vi "align single wall angleV1.0.vi"(8 "error in (no error)":errorcluster, 9 "gyro degree":dbl, 10 "dir":bool, 11 "Target Voltage":dbl) -> (0 "Error Out":errorcluster)   [LabVIEW 2019]
uses:
  <vilib>/Platform/TimedLoop/XDataNode/timing_clust.ctl
  <vilib>/Platform/TimedLoop/XDataNode/nitl_modes.ctl
  <vilib>/Platform/TimedLoop/XDataNode/wakeup.ctl
  <vilib>/addons/control/pid/pid.llb/PID (DBL).vi
  <vilib>/platform/TimedLoop/XDataNode/XDataNode.xnode
  <vilib>/Platform/TimedLoop/XDataNode/XDNodeRunTimeDep.lvlib
  <vilib>/addons/control/pid/NI_PID_pid.lvlib
panel:
  out "Waveform Chart 2":dbl(graph)
  out "Waveform Chart":dbl(graph)
  in  "skip IR":bool
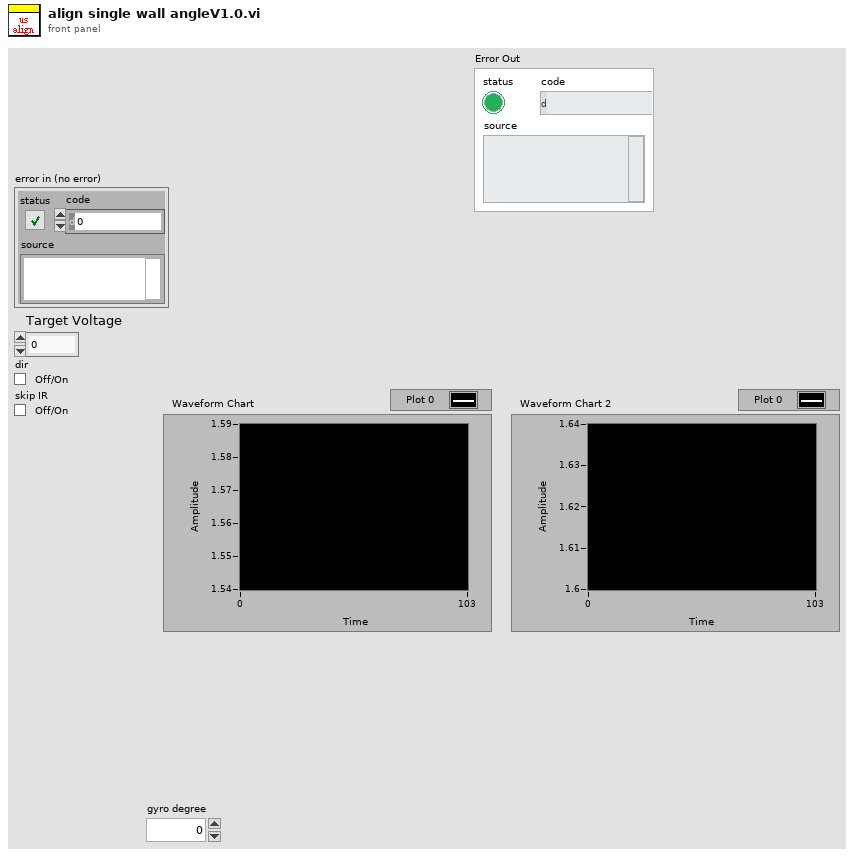
[diagram p1: front panel]
types:
  T1 = typedef "XDNodeRunTimeDep.lvlib/timing_clust.ctl" = cluster{"Expected End [f-1]":u64, "Actual End [f-1]":u64, "Finished Late? [f-1]":bool, "Expected End [i-1]":u64, "Actual End [i-1]":u64, "Finished Late? [i-1]":bool, "Expected Start [i]":u64, "Actual Start [i]":u64, "Expected Start [f]":u64, "Actual Start [f]":u64, "Source Name":string, "Structure Name":string, "Period":i64, "Deadline":i64, "Offset":i64, "Start":i64, "Priority":i32, "Timeout":i32, "Mode":T2, "Wakeup Reason":T3, "Error":errorcluster, "Source Type":string, "Secondary Source Type":string, "Global End Time":u64, "Global Start Time":u64, "Frame Duration":u64, "Iteration Duration":u64, "Assigned CPU":i32, "I/O Scan Engine Mode":u32}
  T2 = typedef "XDNodeRunTimeDep.lvlib/nitl_modes.ctl" = enum32{"No Change", "Process missed periods, maintain original phase", "Discard missed periods, maintain original phase", "Process missed periods, ignore original phase", "Discard missed periods, ignore original phase"}
  T3 = typedef "XDNodeRunTimeDep.lvlib/wakeup.ctl" = enum32{"Normal", "Aborted", "Asynchronous wakeup", "Timing source error", "Timed loop error", "Timeout"}
  T4 = typedef "IR out.ctl" = cluster{"DC estimate (V) 2":dbl, "DC estimate (V)":dbl, "AC estimate (Vrms)":dbl, "AC estimate (Vrms) 2":dbl}
  T5 = cluster{"dbl Scaled Value":dbl, "dbl Scaled Value":dbl}
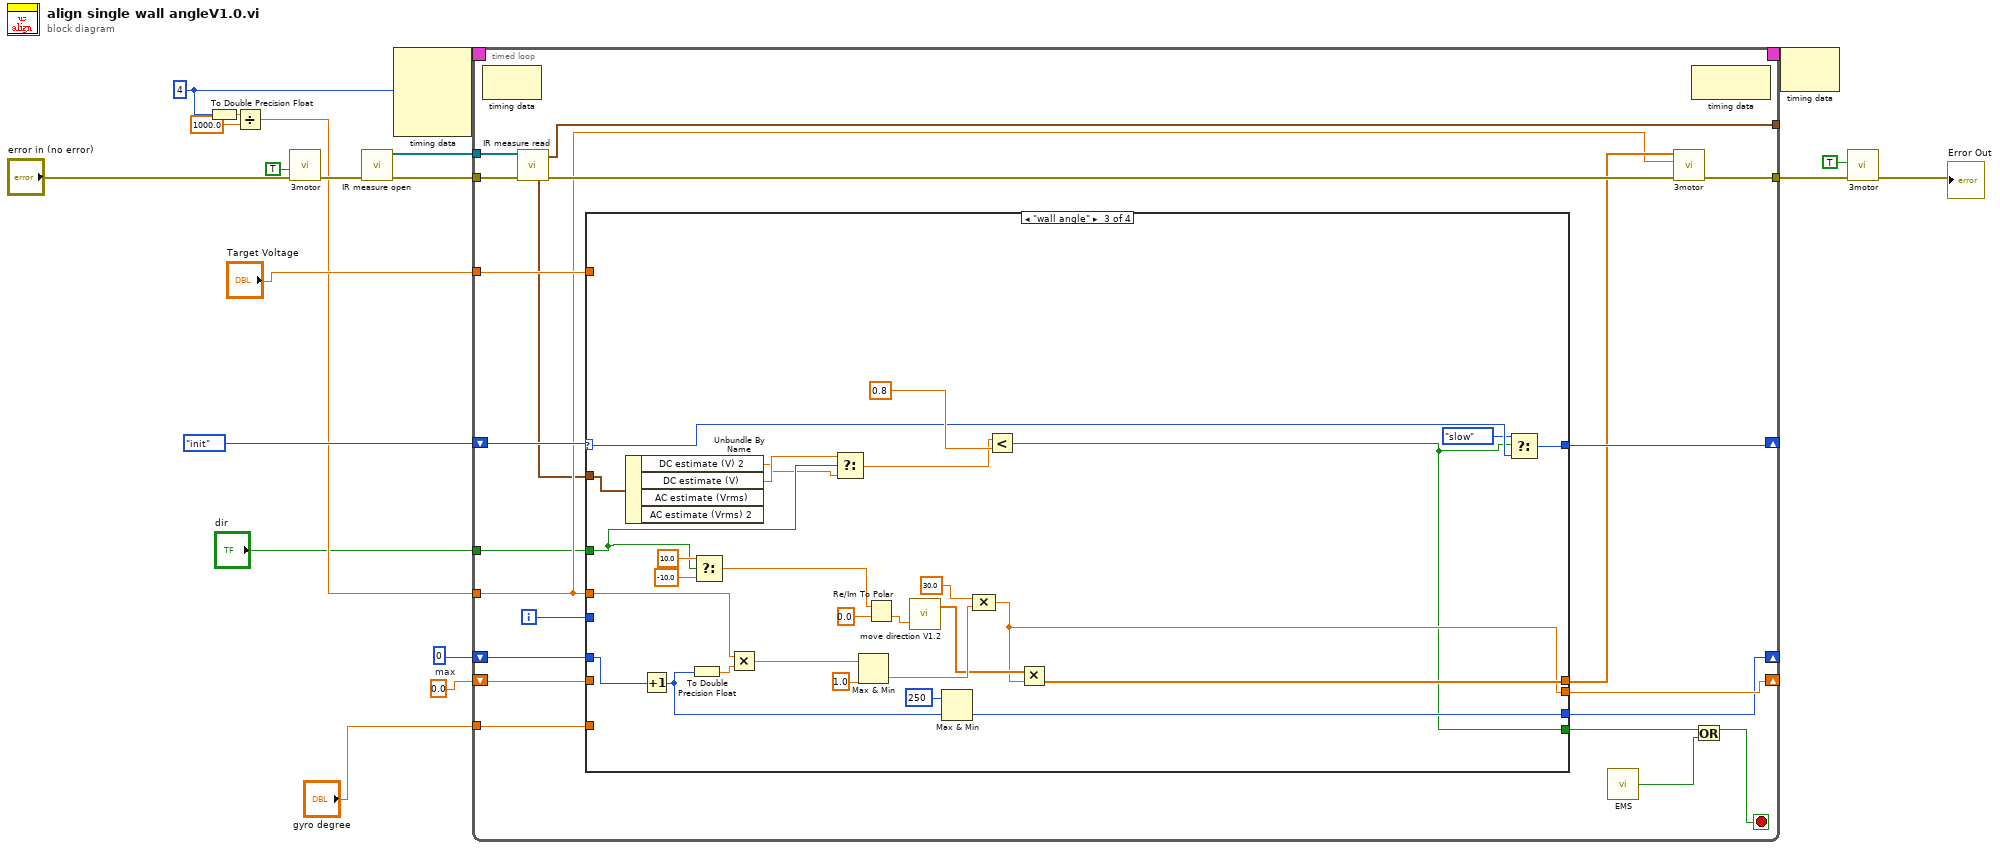
[diagram p0: block diagram]
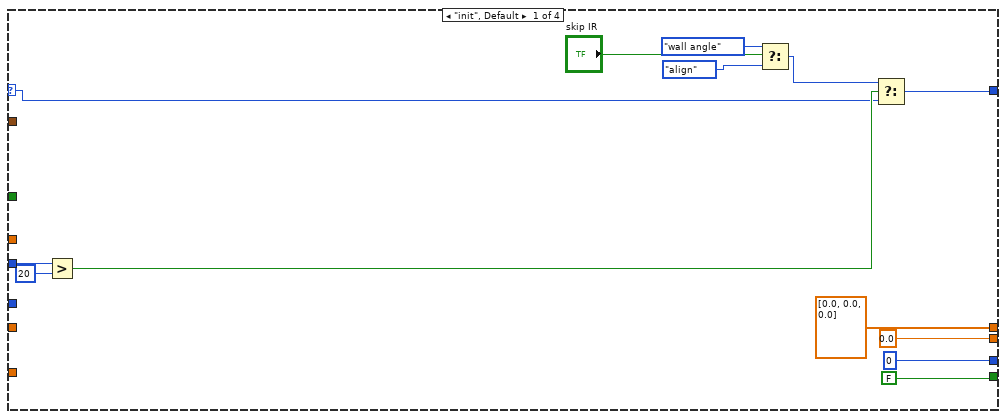
[diagram p2: hidden frame]
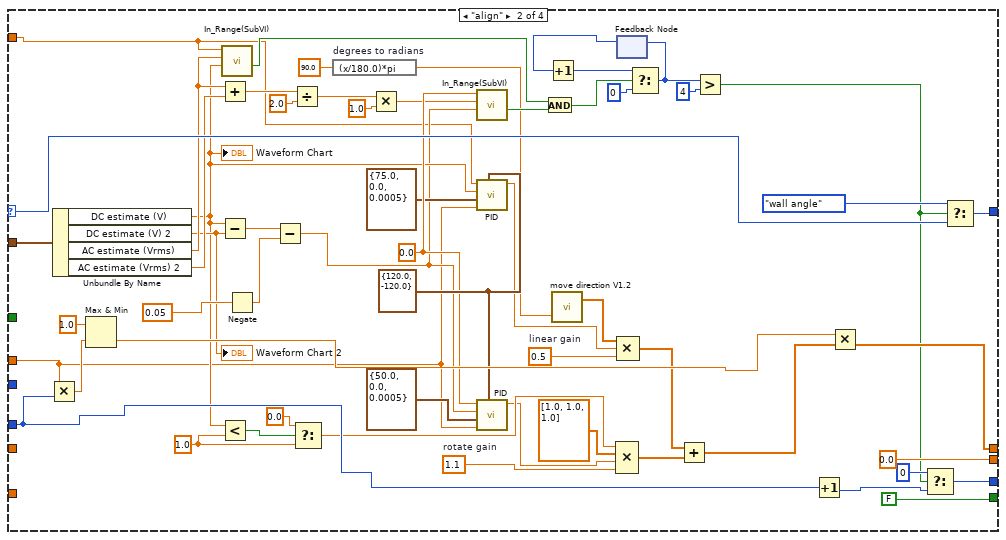
[diagram p3: hidden frame]
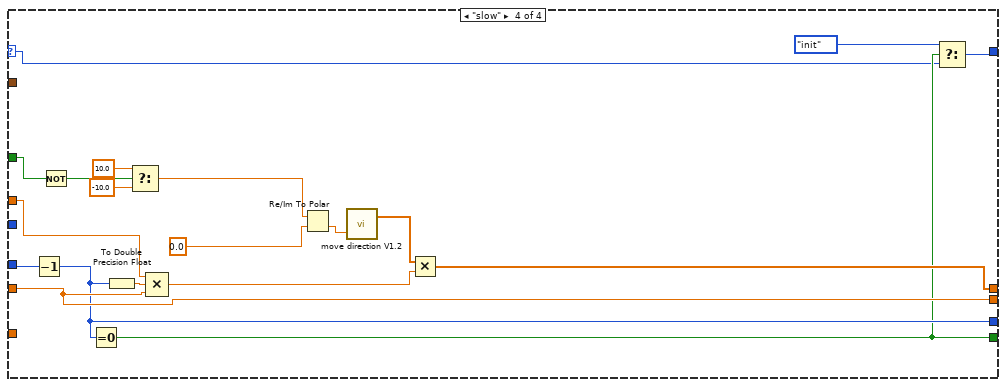
[diagram p4: hidden frame]
diagram:
  w4 = 0.0  # max
  w9 = i64 4 ("Period")
  n1 = To Double Precision Float(number=w9) -> (double precision float=w7:dbl)
  n2 = Divide(x=w7, y=1000.0) -> (x/y=w6:dbl)
  n3 = call "3motor.vi"("error in (no error)"="error in (no error)", "Reset"=TRUE) -> ("error out"=w15:errorcluster)  [unwired: 8 in, 1 out]
  n4 = call "IR measure open.vi"("error in (no error)"=w15) -> ("error out"=w17:errorcluster, "ref array"=w18:refnum<class "IR sensor.lvclass">[])  [unwired: 9 in]
  n5 = node-c288(w9) -> (w20:T1)  [unwired: 3 in]
  n6 = timed-loop {
    timing: w20 -> [_]
    timing-out: [_] -> w19
    tunnel: w18 -> [w41]
    tunnel: w17 -> [w40]
    shift-right: [w38] -> _
    shift-left: enum16{"init", "align", "wall angle", "slow"}."init" -> [w39]
    tunnel: [w36] -> w11
    tunnel: "Target Voltage" -> [w35]
    tunnel: w6 -> [w33]
    tunnel: "dir" -> [w32]
    shift-right: [w30] -> _
    shift-left: w4 -> [w31]
    shift-right: [w28] -> _
    shift-left: 0 -> [w29]
    tunnel: [w24] -> _
    tunnel: "gyro degree" -> [w23]
    i -> [w22]
    stop <- w26 stop-if-true
    n7 = node-c288() -> ()  [unwired: 1 in, 1 out]
    n8 = call "IR measure read.vi"("error in (no error)"=w40, "ref array"=w41) -> ("error out"=w37:errorcluster, "output cluster"=w21:T4, "Waveform Chart"=w24:T5)  [unwired: 7 in]
    n9 = case shown="\"wall angle\"" w39 {
      selector: w39 -> [w51 w110 w125 w146]
      tunnel: w22 -> [w54 _ _ _]
      tunnel: [w50 w111 w126 w144] -> w38
      tunnel: w35 -> [_ w57 _ _]
      tunnel: w33 -> [_ w56 w137 w143]
      tunnel: [dbl[] [0.0, 0.0, 0.0] w100 w129 w150] -> w34
      tunnel: w32 -> [_ _ w114 w154]
      tunnel: w31 -> [_ _ _ w149]
      tunnel: [0.0 0.0 w127 w149] -> w30
      tunnel: w29 -> [_ w101 w123 w158]
      tunnel: [0 w104 w121 w148] -> w28
      tunnel: [FALSE FALSE w119 w147] -> w27
      tunnel: w23 -> [_ _ _ _]
      tunnel: w21 -> [_ w55 w118 _]
      frame "init", Default {
        n10 = Greater?(x=w54, y=20) -> (0:w52:bool)
        n11 = Select(t=enum16{"init", "align", "wall angle", "slow"}."wall angle", s="skip IR", f=enum16{"init", "align", "wall angle", "slow"}."align" ("t")) -> (s? t:f=w45:enum16{"init", "align", "wall angle", "slow"})
        n12 = Select(t=w45, s=w52, f=w51) -> (s? t:f=w50:enum16{"init", "align", "wall angle", "slow"})
      }
      frame "align" {
        w74 = 1.0 ("y")
        w98 = 0.5  # linear gain
        w87 = 1.1  # rotate gain
        w95 = 0.0 ("Setpoint")
        w97 = cluster{"output high":dbl, "output low":dbl} {"output high"=120.0, "output low"=-120.0} ("output range")
        n13 = Multiply(x=w56, y=w101) -> (x*y=w106:dbl)
        n14 = Unbundle By Name(w55) -> ("DC estimate (V)"=w68:dbl, "DC estimate (V) 2"=w80:dbl, "AC estimate (Vrms)"=w94:dbl, "AC estimate (Vrms) 2"=w93:dbl)
        "Waveform Chart" <- w68
        "Waveform Chart 2" <- w80
        n15 = Max & Min(x=1.0, y=w106) -> (min(x,y)=w99:dbl)  [unwired: 1 out]
        n16 = Add(x=w94, y=w93) -> (x+y=w92:dbl)
        n17 = Subtract(x=w68, y=w80) -> (x-y=w64:dbl)
        n18 = Less?(x=w68, y=w74) -> (x < y?=w76:bool)
        n19 = call "In_Range(SubVI).vi"("Proccess Variable"=w68, "AC estimate (Vrms)"=w94, "Setpoint"=w57) -> ("In Range?"=w79:bool)  [unwired: 7 in, 1 out]
        n20 = Negate(x=0.05 ("align offset")) -> (-x=w63:dbl)
        n21 = Subtract(x=w64, y=w63) -> (x-y=w65:dbl)
        n22 = Divide(x=w92, y=2.0) -> (x/y=w90:dbl)
        n23 = Select(t=0.0, s=w76, f=w74) -> (s? t:f=w73:dbl)
        n24 = expression code="(x/180.0)*pi" "degrees to radians"(90.0) -> (w61:dbl)
        n25 = Multiply(x=w90, y=1.0) -> (x*y=w72:dbl)
        n26 = call "In_Range(SubVI).vi"("Proccess Variable"=w65, "AC estimate (Vrms)"=w72, "Setpoint"=w95) -> ("In Range?"=w78:bool)  [unwired: 7 in, 1 out]
        n27 = call-poly <vilib>:"PID.vi"("output range"=w97, "dt (s)"=w56, "PID gains"=cluster{"Kp":dbl, "Ki":dbl, "Kd":dbl} {"Kp"=75.0, "Ki"=0.0, "Kd"=0.0005} ("PID"), "process variable"=w68, "setpoint"=w57) -> ("output"=w67:dbl)  [unwired: 5 in, 1 out]
        n28 = call-poly <vilib>:"PID.vi"("output range"=w97, "dt (s)"=w56, "PID gains"=cluster{"Kp":dbl, "Ki":dbl, "Kd":dbl} {"Kp"=50.0, "Ki"=0.0, "Kd"=0.0005} ("PID"), "process variable"=w65, "setpoint"=w95) -> ("output"=w66:dbl)  [unwired: 5 in, 1 out]
        n29 = And(x=w79, y=w78) -> (x .and. y?=w77:bool)
        n30 = call "move direction V1.2.vi"("theta"=w61) -> ("out array"=w60:dbl[])  [unwired: 1 in, 1 out]
        n31 = Compound Arithmetic op=MULTIPLY(w73, dbl[] [1.0, 1.0, 1.0], w66, w87) -> (w85:dbl[])
        n32 = feedback #1() -> (w83:i32)  [unwired: 1 in]
        n33 = Increment(x=w83) -> (x+1=w84:i32)
        n34 = Compound Arithmetic op=MULTIPLY(w60, w67, w98) -> (w86:dbl[])
        n35 = Select(t=w84, s=w77, f=0) -> (s? t:f=w82:i32)
        n36 = feedback-in #1(w82) -> ()
        n37 = Add(x=w86, y=w85) -> (x+y=w58:dbl[])
        n38 = Greater?(x=w82, y=4) -> (0:w59:bool)
        n39 = Increment(x=w101) -> (x+1=w103:i32)
        n40 = Multiply(x=w99, y=w58) -> (x*y=w100:dbl[])
        n41 = Select(t=0, s=w59, f=w103) -> (s? t:f=w104:i32)
        n42 = Select(t=enum16{"init", "align", "wall angle", "slow"}."wall angle", s=w59, f=w110) -> (s? t:f=w111:enum16{"init", "align", "wall angle", "slow"})
      }
      frame "wall angle" {
        n43 = Unbundle By Name(w118) -> ("DC estimate (V) 2"=w112:dbl, "DC estimate (V)"=w113:dbl)  [unwired: 2 out]
        n44 = Increment(x=w123) -> (x+1=w122:i32)
        n45 = To Double Precision Float(number=w122) -> (double precision float=w138:dbl)
        n46 = Select(t=10.0, s=w114, f=-10.0) -> (s? t:f=w117:dbl)
        n47 = Multiply(x=w137, y=w138) -> (x*y=w136:dbl)
        n48 = Select(t=w113, s=w114, f=w112) -> (s? t:f=w115:dbl)
        n49 = Max & Min(x=w136, y=1.0) -> (min(x,y)=w130:dbl)  [unwired: 1 out]
        n50 = Re/Im To Polar(2:0.0 ("y"), 3:w117) -> (0:w132:dbl)  [unwired: 1 out]
        n51 = call "move direction V1.2.vi"("theta"=w132) -> ("out array"=w128:dbl[])  [unwired: 1 in, 1 out]
        n52 = Max & Min(x=250, y=w122) -> (min(x,y)=w121:i32)  [unwired: 1 out]
        n53 = Compound Arithmetic op=MULTIPLY(30.0, w130) -> (w127:dbl)
        n54 = Less?(x=w115, y=0.8 ("x")) -> (x < y?=w119:bool)
        n55 = Multiply(x=w128, y=w127) -> (x*y=w129:dbl[])
        n56 = Select(t=enum16{"init", "align", "wall angle", "slow"}."slow", s=w119, f=w125) -> (s? t:f=w126:enum16{"init", "align", "wall angle", "slow"})
      }
      frame "slow" {
        n57 = Decrement(x=w158) -> (x-1=w148:i32)
        n58 = Not(x=w154) -> (.not. x?=w142:bool)
        n59 = Equal To 0?(x=w148) -> (x = 0?=w147:bool)
        n60 = To Double Precision Float(number=w148) -> (double precision float=w153:dbl)
        n61 = Select(t=10.0, s=w142, f=-10.0) -> (s? t:f=w140:dbl)
        n62 = Compound Arithmetic op=MULTIPLY(w143, w153, w149) -> (w151:dbl)
        n63 = Re/Im To Polar(2:0.0 ("y"), 3:w140) -> (0:w155:dbl)  [unwired: 1 out]
        n64 = call "move direction V1.2.vi"("theta"=w155) -> ("out array"=w152:dbl[])  [unwired: 1 in, 1 out]
        n65 = Multiply(x=w152, y=w151) -> (x*y=w150:dbl[])
        n66 = Select(t=enum16{"init", "align", "wall angle", "slow"}."init", s=w147, f=w146) -> (s? t:f=w144:enum16{"init", "align", "wall angle", "slow"})
      }
    }
    n67 = call "EMS.vi"() -> ("A/DIO4 (Pin 19)"=w25:bool)
    n68 = call "3motor.vi"("error in (no error)"=w37, "dt(s)"=w33, "Motor speed"=w34) -> ("error out"=w36:errorcluster)  [unwired: 7 in, 1 out]
    n69 = node-c288() -> ()  [unwired: 1 in, 1 out]
    n70 = Or(x=w27, y=w25) -> (x .or. y?=w26:bool)
  }
  n71 = node-c288(w19) -> ()  [unwired: 1 out]
  n72 = call "3motor.vi"("error in (no error)"=w11, "Reset"=TRUE) -> ("error out"=→"Error Out":errorcluster)  [unwired: 8 in, 1 out]
